vi "NI VeriStand - Set Item Description.vi"(8 "error in (no error)":errorcluster, 10 "Description":string, 11 "Item Ref in":T1 format="%.0x") -> (0 "error out":errorcluster, 3 "Item Ref out":T1 format="%.0x", 4 "Found":bool)   [LabVIEW 2026, in "Custom Devices Storage.lvlib"]
uses:
  Custom Devices Storage.lvlib
  <vilib>/NI VeriStand/Custom Device API/Custom Device Item Ref.ctl
  C:/Users/Administrator/Desktop/Jatin/All DNC DLLs/NationalInstruments.VeriStand.SystemDefinitionAPI.dll
  Jatin/All DNC DLLs/NationalInstruments.VeriStand.SystemDefinitionAPI.dll
  <vilib>/NI VeriStand/Custom Device API/Custom Device API.lvlib
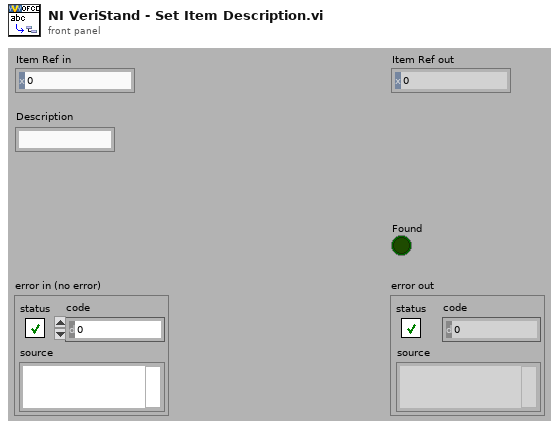
[diagram p1: front panel]
types:
  T1 = typedef "Custom Device API.lvlib/Custom Device Item Ref.ctl" = u64
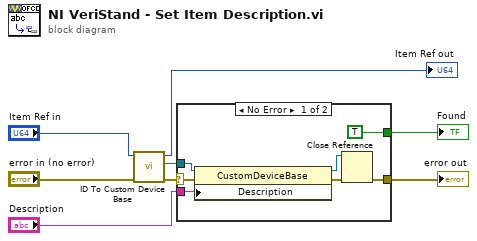
[diagram p0: block diagram]
diagram:
  n1 = call "ID To Custom Device Base.vi"("error in (no error)"="error in (no error)", "ID in"="Item Ref in") -> ("error out"=w5:errorcluster, "NationalInstruments.VeriStand.SystemDefinitionAPI.CustomDeviceBase"=w4:refnum<k39>, "ID out"=→"Item Ref out":u64)  [unwired: 7 in]
  n2 = case shown="No Error" w5 {
    selector: w5 -> [w13 w16]
    tunnel: w4 -> [w15 _]
    tunnel: "Description" -> [w14 _]
    tunnel: [w10 w16] -> w2
    tunnel: [TRUE _] -> w1
    frame No Error {
      n3 = property class="CustomDeviceBase"(reference=w15, error in=w13, "Description"=w14) -> (reference out=w12:refnum<k39>, error out=w11:errorcluster)
      n4 = Close Reference(reference=w12, error in (no error)=w11) -> (error out=w10:errorcluster)
    }
    frame Error {
    }
  }
  "error out" <- w2
  "Found" <- w1
